vi "TypeDescriptor_GetUnits.vi"(11 "type descriptor":i16[](array[numeric]) format="%.0x") -> (1 "has Units":bool, 2 "Units":T1[](array[typedef]), 3 "type descriptor dup":i16[](array[numeric]) format="%.0x")   [LabVIEW 2013, in "OpenDescriptor.lvlib"]
uses:
  OpenDescriptor.lvlib
  <vilib>/Utility/VariantDataType/UnitInfo.ctl
  <vilib>/Utility/VariantDataType/UnitType.ctl
  <vilib>/Utility/VariantDataType/VariantType.lvlib
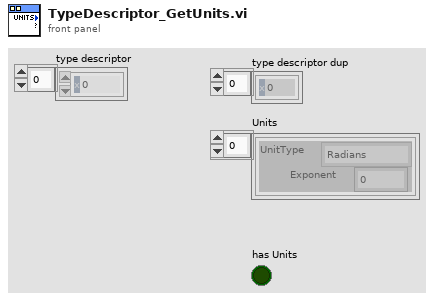
[diagram p1: front panel]
types:
  T1 = typedef "VariantType.lvlib/UnitInfo.ctl" = cluster{"UnitType":T2, "Exponent":i16}
  T2 = typedef "VariantType.lvlib/UnitType.ctl" = enum16{"Radians", "Steradians", "Seconds", "Meters", "Kilograms", "Amperes", "Kelvins", "Moles", "Candelas", "InvalidUnit"}
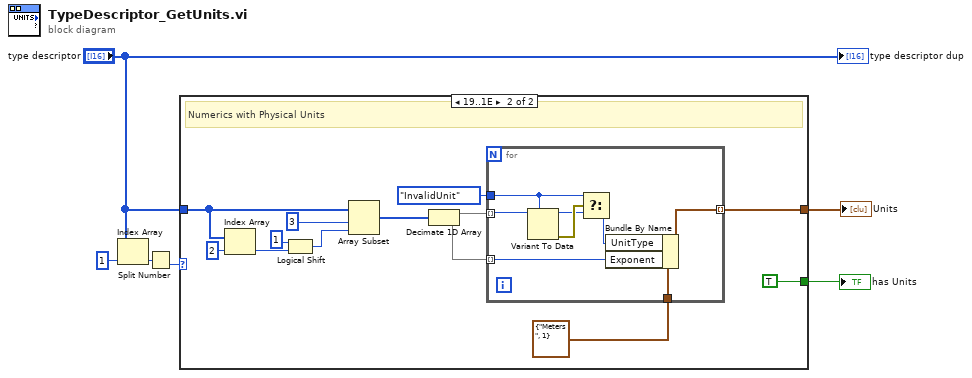
[diagram p0: block diagram]
diagram:
  n1 = Index Array(array="type descriptor", index=1) -> (element=w5:i16)
  n2 = Split Number(x=w5) -> (lo(x)=w2:u8)  [unwired: 1 out]
  n3 = case shown="19..1E" w2 {
    tunnel: [_ w8] -> w6
    tunnel: "type descriptor" -> [_ w16]
    tunnel: [_ TRUE] -> w1
    frame Default {
      # "No Units"
    }
    frame 25..30 {
      # "Numerics with Physical Units"
      n4 = Index Array(array=w16, index=2) -> (element=w17:i16)
      n5 = Logical Shift(y=i16 1, x=w17) -> (x << y=w14:i16)
      n6 = Array Subset(array=w16, index=3, length=w14) -> (w13:i16[])
      n7 = Decimate 1D Array(w13) -> (w12:i16[], w11:i16[])
      n8 = for {
        tunnel: w12 -> [w27] mode=indexing
        tunnel: w11 -> [w21] mode=indexing
        tunnel: UnitType."InvalidUnit" ("UnitType") -> [w24]
        tunnel: T1 {"UnitType"=enum."Meters", "Exponent"=1} ("Unit") -> [w23]
        tunnel: [w20] -> w8 mode=indexing
        n9 = Variant To Data(type=w24, Variant=w27) -> (data=w25:T2, error out=w26:errorcluster)  [unwired: 1 in]
        n10 = Select(t=w24, s=w26, f=w25) -> (s? t:f=w22:T2)
        n11 = Bundle By Name(cluster=w23, "UnitType"=w22, "Exponent"=w21) -> (w20:T1)
      }
    }
  }
  "Units" <- w6
  "has Units" <- w1
  "type descriptor dup" <- "type descriptor"
